vi "Read aVar Params.vi"(8 "error in":errorcluster, 11 "CRDS Cell in":refnum<class "CRDS Cell.lvclass">) -> (0 "error out":errorcluster, 2 "aVar Params":T1={"tmeas"=0.001, "tint"=[0.001, 0.01, 0.1, 1.0, 3.0], "ttot"=15.0, "Varaince On"=FALSE}, 3 "CRDS Cell out":refnum<class "CRDS Cell.lvclass">)   [LabVIEW 2012, in "CRDS Cell.lvclass"]
uses:
  CRDS Cell.lvclass
  CRDS Cell.lvclass/CRDS Cell.ctl
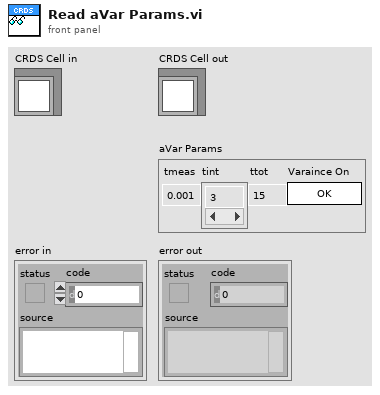
[diagram p1: front panel]
types:
  T1 = cluster{"tmeas":dbl, "tint":sgl[], "ttot":dbl, "Varaince On":bool}
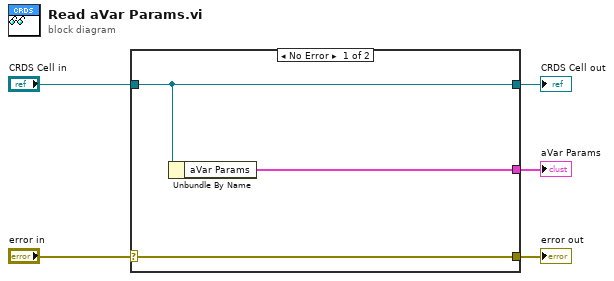
[diagram p0: block diagram]
diagram:
  n1 = case shown="No Error" "error in" {
    selector: "error in" -> [w8 w9]
    tunnel: [w8 w9] -> w4
    tunnel: [w7 w10] -> w2
    tunnel: "CRDS Cell in" -> [w7 w10]
    tunnel: [w6 _] -> w1
    frame No Error {
      n2 = Unbundle By Name(w7) -> ("aVar Params"=w6:T1)
    }
    frame Error {
    }
  }
  "error out" <- w4
  "CRDS Cell out" <- w2
  "aVar Params" <- w1
